vi "TestPasse3PeacesOfField.vi"(10 "Field Length":u32, 11 "X":dbl format="%#_13g") -> (1 "Terceiro Terço":bool=TRUE, 2 "Segundo Terço":bool=TRUE, 3 "Primeiro Terço":bool=TRUE)   [LabVIEW 2017]
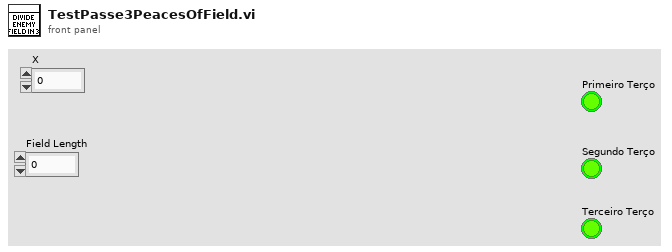
[diagram p1: front panel]
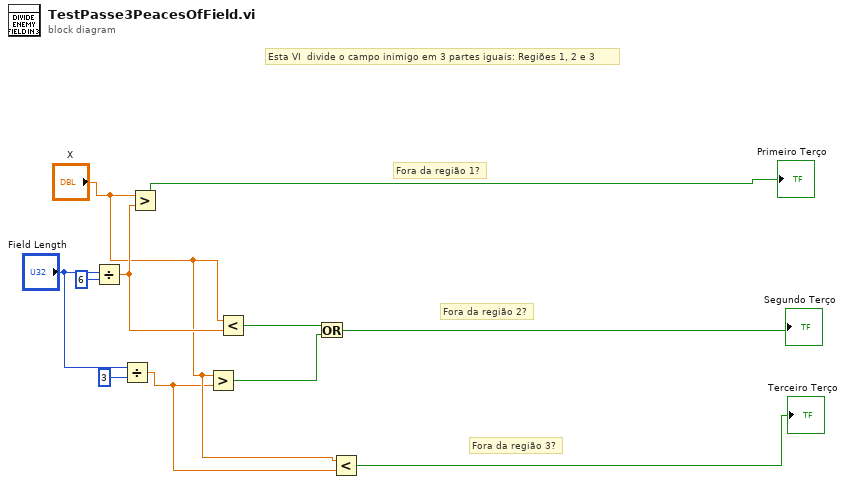
[diagram p0: block diagram]
diagram:
  # "Esta VI  divide o campo inimigo em 3 partes iguais: Regiões 1, 2 e 3"
  # "Fora da região 3?"
  # "Fora da região 2?"
  # "Fora da região 1?"
  n1 = Divide(x="Field Length", y=6) -> (x/y=w9:dbl)
  n2 = Divide(x="Field Length", y=3) -> (x/y=w2:dbl)
  n3 = Greater?(x="X", y=w9) -> (0:→"Primeiro Terço":bool)
  n4 = Greater?(x="X", y=w2) -> (0:w4:bool)
  n5 = Less?(x="X", y=w9) -> (x < y?=w7:bool)
  n6 = Or(x=w7, y=w4) -> (x .or. y?=→"Segundo Terço":bool)
  n7 = Less?(x="X", y=w2) -> (x < y?=→"Terceiro Terço":bool)
